vi "Brower View Get Item Symbol.vi"(8 "error in (no error)":errorcluster, 11 "Brower View in":refnum<class "Brower View.lvclass">) -> (0 "error out":errorcluster, 2 "Symbol":i32, 3 "Brower View out":refnum<class "Brower View.lvclass">)   [LabVIEW 2015, in "Brower View.lvclass"]
uses:
  Brower View.lvclass
  Brower View.lvclass/Brower View.ctl
  MyTreeAPI/MyTreeAPI.lvclass
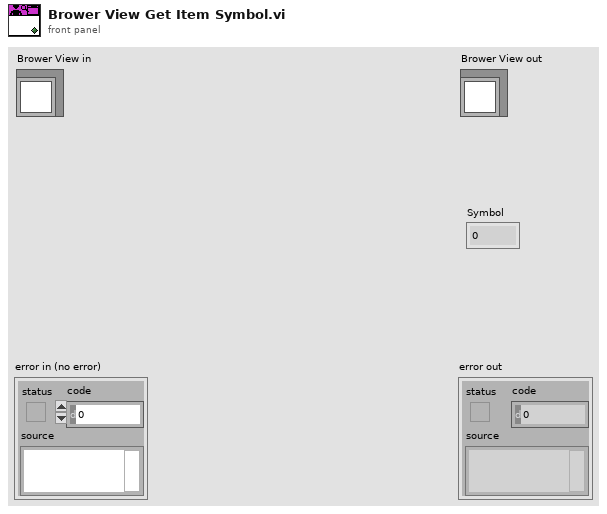
[diagram p1: front panel]
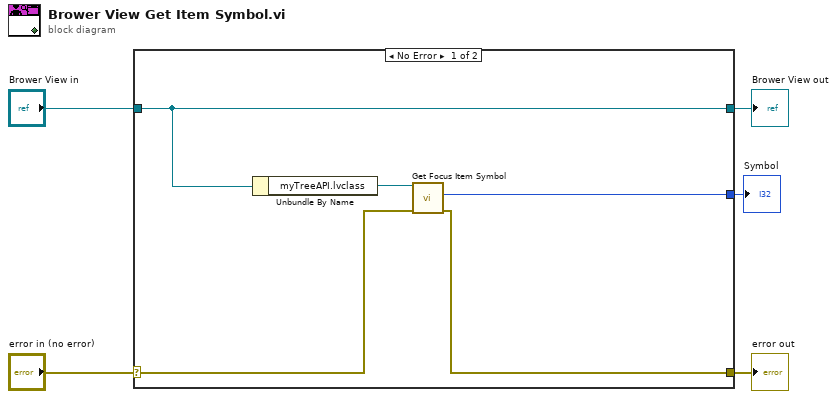
[diagram p0: block diagram]
diagram:
  n1 = case shown="No Error" "error in (no error)" {
    selector: "error in (no error)" -> [w8 w12]
    tunnel: [w7 w12] -> w4
    tunnel: [w10 w11] -> w2
    tunnel: "Brower View in" -> [w10 w11]
    tunnel: [w6 _] -> w1
    frame No Error {
      n2 = Unbundle By Name(w10) -> ("myTreeAPI.lvclass"=w9:refnum<class "MyTreeAPI.lvclass">)
      n3 = call "Get Focus Item Symbol.vi"("error in (no error)"=w8, "MyTreeAPI in"=w9) -> ("error out"=w7:errorcluster, "Symbol"=w6:i32)  [unwired: 7 in, 1 out]
    }
    frame Error {
    }
  }
  "error out" <- w4
  "Brower View out" <- w2
  "Symbol" <- w1
